vi "Test Next Interval.vi"() -> ()   [LabVIEW 2021, in "Interval Timer.lvlib"]
doc: "Test the behavior of Next Interval.vi."
uses:
  Interval Timer.lvlib
  Repeat Interval.ctl
  Interval Length.ctl
  Interval Token.ctl
panel:
  out "message":string
  in  "stop":bool
  out "Interval Token out":T1
  in  "Intervals in":T2[](array[typedef])=[{"Interval"=enum."10 seconds", "Count"=10}]
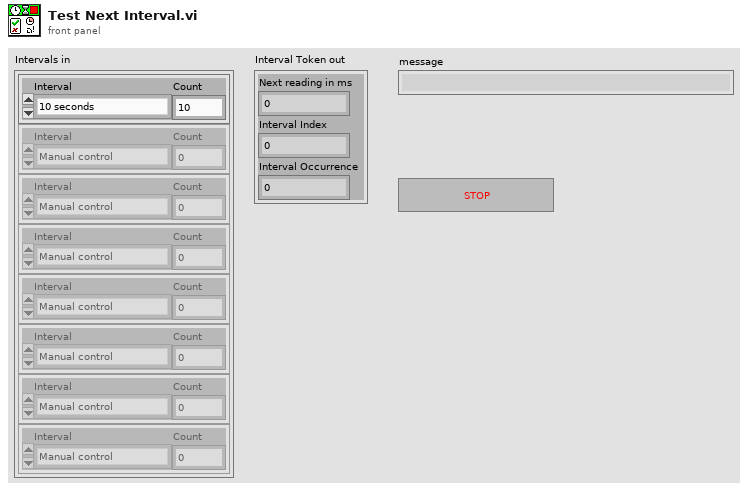
[diagram p1: front panel]
types:
  T1 = typedef "Interval Timer.lvlib/Interval Token.ctl" = cluster{"Next reading in ms":u32, "Interval Index":i32, "Interval Occurrence":i32}
  T2 = typedef "Interval Timer.lvlib/Repeat Interval.ctl" = cluster{"Interval":T3, "Count":i32}
  T3 = typedef "Interval Timer.lvlib/Interval Length.ctl" = enum16{"Manual control", "1 second", "10 seconds", "30 seconds", "60 seconds", "600 seconds", "1200 seconds", "3600 seconds"}
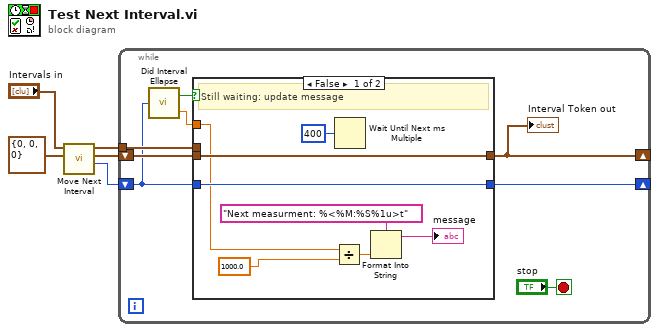
[diagram p0: block diagram]
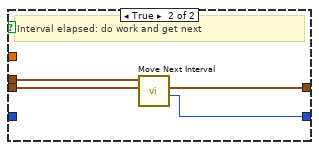
[diagram p2: hidden frame]
diagram:
  n1 = call "Move Next Interval.vi"("Interval Token in"=T1 {"Next reading in ms"=0, "Interval Index"=0, "Interval Occurrence"=0}, "Intervals in"="Intervals in") -> ("Next interval time (ms)"=w5:u32, "Interval Token out"=w1:T1, "Intervals out"=w2:T2[])  [unwired: 6 in, 1 out]
  n2 = while {
    tunnel: w2 -> [w13]
    shift-right: [w10] -> _
    shift-left: w1 -> [w12]
    shift-right: [w8] -> _
    shift-left: w5 -> [w7]
    stop <- "stop" stop-if-true
    n3 = call "Did Interval Ellapse.vi"("Future time coordinate (ms)"=w7) -> ("ms Until Next"=w6:dbl, "Interval Ellapsed?"=w9:bool)  [unwired: 2 in]
    n4 = case shown="False" w9 {
      tunnel: w13 -> [_ w25]
      tunnel: w12 -> [w15 w24]
      tunnel: [w16 w23] -> w8
      tunnel: [w15 w22] -> w10
      tunnel: w7 -> [w16 _]
      tunnel: w6 -> [w14 _]
      frame False {
        # "Still waiting: update message"
        n5 = Divide(x=w14, y=1000.0) -> (x/y=w20:dbl)
        n6 = Wait Until Next ms Multiple(millisecond multiple=u32 400) -> ()  [unwired: 1 out]
        n7 = Format Into String(format string="Next measurment: %<%M:%S%1u>t", w20) -> (resulting string=→"message":string)  [unwired: 2 in, 1 out]
      }
      frame True {
        # "Interval elapsed: do work and get next"
        n8 = call "Move Next Interval.vi"("Interval Token in"=w24, "Intervals in"=w25) -> ("Next interval time (ms)"=w23:u32, "Interval Token out"=w22:T1)  [unwired: 6 in, 2 out]
      }
    }
    "Interval Token out" <- w10
  }
